vi "Right Gripper Open.vi"(6 "Delay":u32=1000, 11 "error in":errorcluster) -> (3 "error out":errorcluster)   [LabVIEW 2013]
uses:
  ROS/Code/SubVIs/BaxterSide.ctl
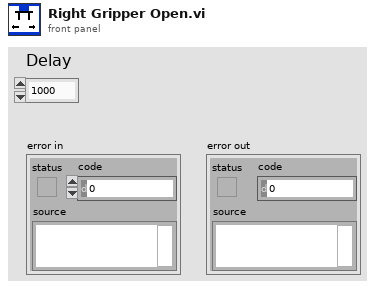
[diagram p1: front panel]
types:
  T1 = typedef "BaxterSide.ctl" = enum16{"left", "right"}
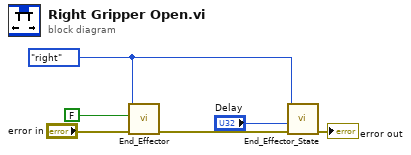
[diagram p0: block diagram]
diagram:
  w2 = BaxterSide."right" ("Side")
  n1 = call "End_Effector.vi"("error in"="error in", "Close"=FALSE ("Open?"), "Side"=w2) -> ("error out"=w6:errorcluster)  [unwired: 5 in]
  n2 = call "End_Effector_State.vi"("error in"=w6, "Delay"="Delay", "Side"=w2) -> ("error out"=→"error out":errorcluster)  [unwired: 2 in, 3 out]
